vi "Read Network Master.vi"(8 "error in":errorcluster, 11 "MB CR in":refnum<class "Modbus Master CR API.lvclass">) -> (0 "error out":errorcluster, 2 "Modbus Master CR":refnum<class "Modbus Master CR.lvclass">, 3 "MB CR out":refnum<class "Modbus Master CR API.lvclass">)   [LabVIEW 2021, in "Modbus Master CR API.lvclass"]
doc: "This VI is an accessor for the function definition stored in the Modbus master instance. This accessor can be used as a property node. This function definition is used by the master to determine how to pack and unpack Modbus protocol data units."
uses:
  Modbus Master CR API.lvclass
  C:/my_projects/projects/Algorithms/Labview/21/Modbus_v121c/API/Modbus API.lvclass
  Modbus API.lvclass/Modbus API.ctl
  Modbus Master CR API.lvclass/Modbus Master CR API.ctl
  Network Protocol/MB/Modbus Master CR.lvclass
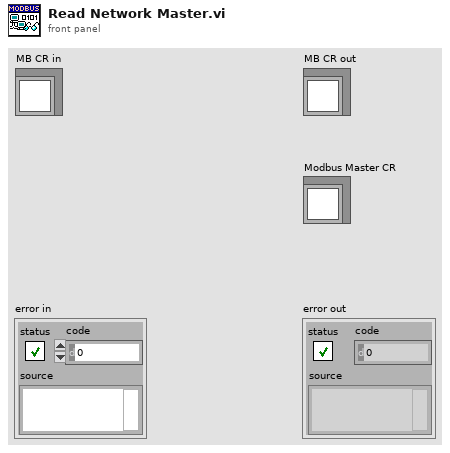
[diagram p1: front panel]
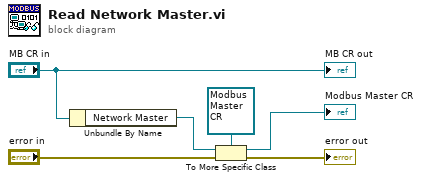
[diagram p0: block diagram]
diagram:
  n1 = Unbundle By Name("MB CR in") -> ("Network Master"=w3:refnum<class "Network Master.lvclass">)
  n2 = To More Specific Class(target class=refnum<class "Modbus Master CR.lvclass"> refnum ("Modbus Master CR.lvclass"), reference=w3, error in="error in") -> (specific class reference=→"Modbus Master CR":refnum<class "Modbus Master CR.lvclass">, error out=→"error out":errorcluster)
  "MB CR out" <- "MB CR in"
